vi "Read Percepcja.vi"(8 "error in (no error)":errorcluster, 11 "Boid in":refnum<class "Boid.lvclass">) -> (0 "error out":errorcluster, 2 "Percepcja":cluster{"Zakres":i16, "Kat":i16}={"Zakres"=30, "Kat"=120}, 3 "Boid out":refnum<class "Boid.lvclass">)   [LabVIEW 2014, in "Boid.lvclass"]
uses:
  Boid.lvclass
  Boid.lvclass/Boid.ctl
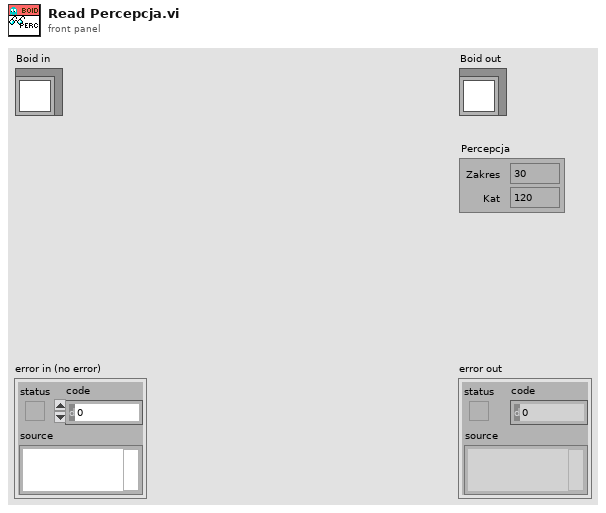
[diagram p1: front panel]
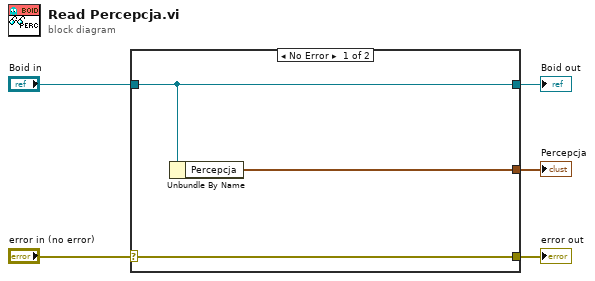
[diagram p0: block diagram]
diagram:
  n1 = case shown="No Error" "error in (no error)" {
    selector: "error in (no error)" -> [w8 w9]
    tunnel: [w8 w9] -> w4
    tunnel: [w7 w10] -> w2
    tunnel: "Boid in" -> [w7 w10]
    tunnel: [w6 _] -> w1
    frame No Error {
      n2 = Unbundle By Name(w7) -> ("Percepcja"=w6:cluster{"Zakres":i16, "Kat":i16})
    }
    frame Error {
    }
  }
  "error out" <- w4
  "Boid out" <- w2
  "Percepcja" <- w1
